vi "Copy Value.vi"(8 "error in (no error)":errorcluster, 10 "From":refnum<class "Type.lvclass">, 11 "Entity Collection in":refnum<class "Entity Collection.lvclass">) -> (0 "error out":errorcluster, 3 "Entity Collection out":refnum<class "Entity Collection.lvclass">)   [LabVIEW 2020, in "Conditum.lvlib" / "Columns.lvlib" / "Entity Collection.lvclass"]
uses:
  Entity Collection.lvclass
  Type/Type.lvclass
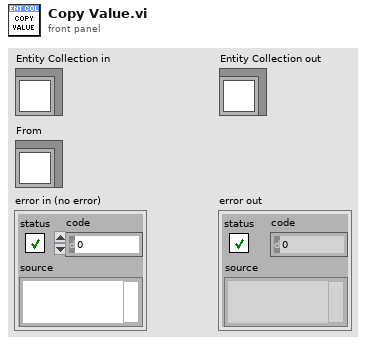
[diagram p1: front panel]
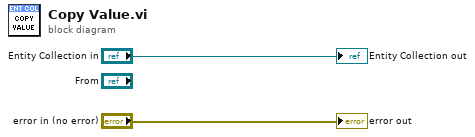
[diagram p0: block diagram]
diagram:
  "error out" <- "error in (no error)"
  "Entity Collection out" <- "Entity Collection in"
